vi "Import - Tx Packet.vi"(7 "Tx Packet":T1 {"Endianness" items=["big-endian"=0, "little-endian"=2]}, 8 "error in (no error)":errorcluster, 11 "Device Item Ref in":T6 format="%.0x") -> (0 "error out":errorcluster)   [LabVIEW 2016, in "UDP-Custom-Device System Explorer.lvlib"]
uses:
  UDP-Custom-Device System Explorer.lvlib
  <vilib>/NI Veristand/Custom Device API/Custom Device Item Ref.ctl
  Types/XML - New/ImpExp - Tx Packet Data.ctl
  <vilib>/NI Veristand/Custom Device API/Custom Device Item Info.ctl
  Shared/Types/Shared - Channel Data Type.ctl
  Shared/Types/Shared - Buffered.PacketInfo.ctl
  Shared/Types/Shared - Pointer Encoding.ctl
  Property Accessors/Shared Packet Accessors.lvlib
  Property Accessors/Tx Packet Accessors.lvlib
  <vilib>/NI VeriStand/Custom Device API/Custom Device API.lvlib
  <vilib>/NI VeriStand/Custom Device Tools/Custom Device Utility Library/Custom Device Utility Library.lvlib
  Shared/UDP-Custom-Device Shared.lvlib
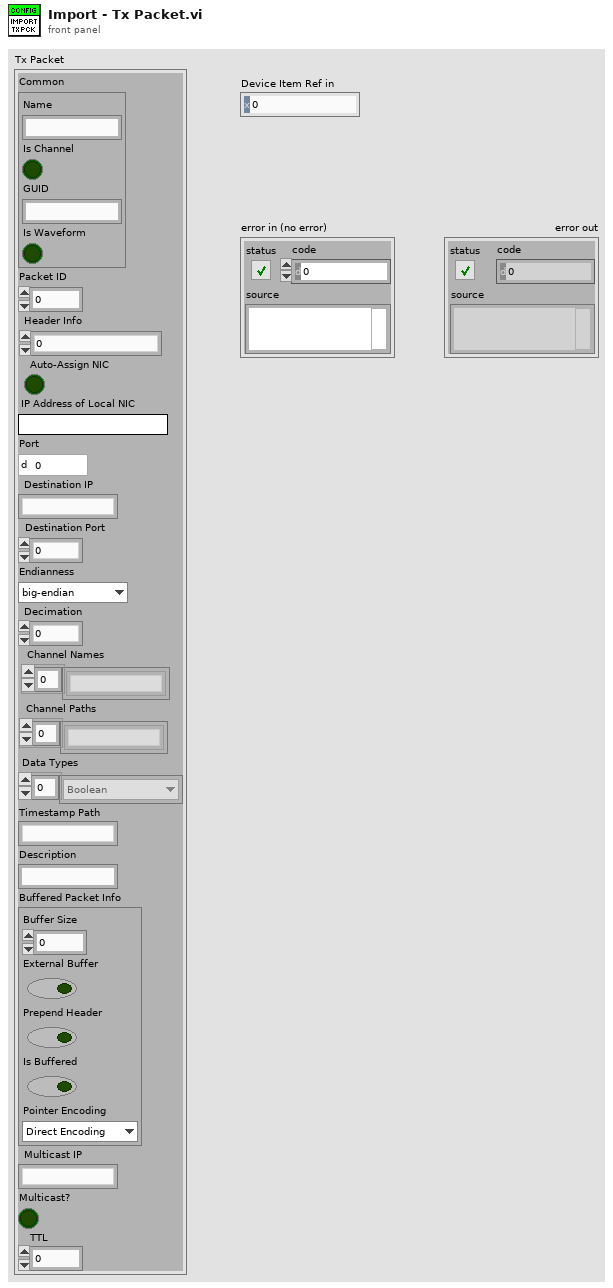
[diagram p1: front panel]
types:
  T1 = typedef "UDP-Custom-Device System Explorer.lvlib/ImpExp - Tx Packet Data.ctl" = cluster{"Common":T2, "Packet ID":i32, "Header Info":u32, "Auto-Assign NIC":bool, "IP Address of Local NIC":string, "Port":u16, "Destination IP":string, "Destination Port":u16, "Endianness":u16, "Decimation":u16, "Channel Names":string[], "Channel Paths":string[], "Data Types":T3[], "Timestamp Path":string, "Description":string, "Buffered Packet Info":T4, "Multicast IP":string, "Multicast?":bool, "TTL":u16}
  T2 = typedef "Custom Device API.lvlib/Custom Device Item Info.ctl" = cluster{"Name":string, "Is Channel":bool, "GUID":string, "Is Waveform":bool}
  T3 = typedef "UDP-Custom-Device Shared.lvlib/Shared - Channel Data Type.ctl" = enum16{"Boolean", "Single", "Double", "I8", "I16", "I32", "I64", "U8", "U16", "U32", "U64"}
  T4 = typedef "UDP-Custom-Device Shared.lvlib/Shared - Buffered.PacketInfo.ctl" = cluster{"Buffer Size":i32, "External Buffer":bool, "Prepend Header":bool, "Is Buffered":bool, "Pointer Encoding":T5}
  T5 = typedef "UDP-Custom-Device Shared.lvlib/Shared - Pointer Encoding.ctl" = enum16{"Direct Encoding", "Conversion Encoding"}
  T6 = typedef "Custom Device API.lvlib/Custom Device Item Ref.ctl" = u64
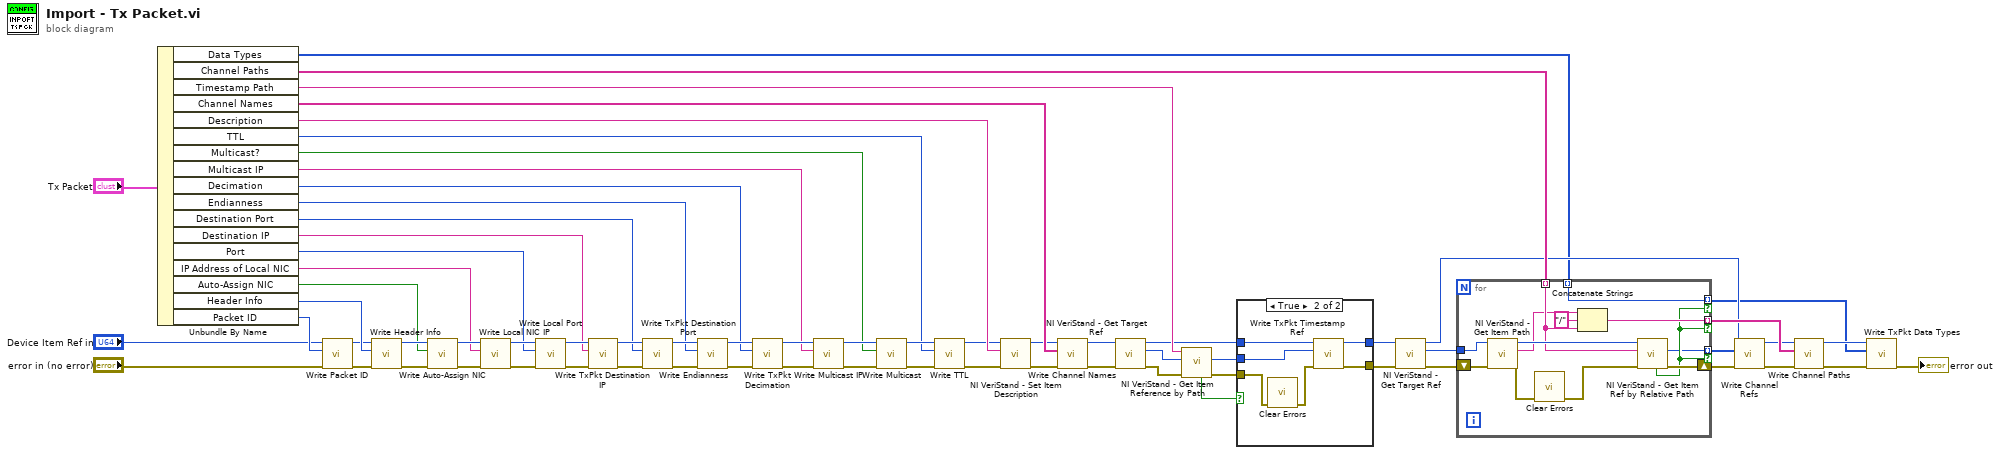
[diagram p0: block diagram]
diagram:
  n1 = Unbundle By Name("Tx Packet") -> ("Data Types"=w16:T3[], "Channel Paths"=w24:string[], "Timestamp Path"=w31:string, "Channel Names"=w39:string[], "Description"=w42:string, "TTL"=w1:u16, "Multicast?"=w2:bool, "Multicast IP"=w3:string, "Decimation"=w43:u16, "Endianness"=w44:u16, "Destination Port"=w49:u16, "Destination IP"=w50:string, "Port"=w51:u16, "IP Address of Local NIC"=w52:string, "Auto-Assign NIC"=w61:bool, "Header Info"=w66:u32, "Packet ID"=w67:i32)
  n2 = call "Write Packet ID.vi"("error in (no error)"="error in (no error)", "Packet ID"=w67, "Node Ptr"="Device Item Ref in") -> ("error out"=w64:errorcluster, "Node Ptr out"=w65:T6)  [unwired: 7 in]
  n3 = call "Write Header Info.vi"("error in (no error)"=w64, "Header Info"=w66, "Node Ptr"=w65) -> ("error out"=w62:errorcluster, "Node Ptr out"=w63:T6)  [unwired: 7 in]
  n4 = call "Write Auto-Assign NIC.vi"("error in (no error)"=w62, "Auto-Assign NIC"=w61, "Node Ptr"=w63) -> ("error out"=w56:errorcluster, "Node Ptr out"=w60:T6)  [unwired: 7 in]
  n5 = call "Write Local NIC IP.vi"("error in (no error)"=w56, "IP Address of Local NIC"=w52, "Node Ptr"=w60) -> ("error out"=w55:errorcluster, "Node Ptr out"=w59:T6)  [unwired: 7 in]
  n6 = call "Write Local Port.vi"("error in (no error)"=w55, "Port"=w51, "Node Ptr"=w59) -> ("error out"=w54:errorcluster, "Node Ptr out"=w58:T6)  [unwired: 7 in]
  n7 = call "Write TxPkt Destination IP.vi"("error in (no error)"=w54, "Destination IP"=w50, "Node Ptr"=w58) -> ("error out"=w53:errorcluster, "Node Ptr out"=w57:T6)  [unwired: 7 in]
  n8 = call "Write TxPkt Destination Port.vi"("error in (no error)"=w53, "Destination Port"=w49, "Node Ptr"=w57) -> ("error out"=w47:errorcluster, "Node Ptr out"=w48:T6)  [unwired: 7 in]
  n9 = call "Write Endianness.vi"("error in (no error)"=w47, "Endianness"=w44, "Node Ptr"=w48) -> ("error out"=w45:errorcluster, "Node Ptr out"=w46:T6)  [unwired: 7 in]
  n10 = call "Write TxPkt Decimation.vi"("error in (no error)"=w45, "Decimation"=w43, "Node Ptr"=w46) -> ("error out"=w11:errorcluster, "Node Ptr out"=w5:T6)  [unwired: 7 in]
  n11 = call "Write Multicast IP.vi"("error in (no error)"=w11, "Multicast IP Address"=w3, "Node Ptr"=w5) -> ("error out"=w10:errorcluster, "Node Ptr out"=w7:T6)  [unwired: 7 in]
  n12 = call "Write Multicast.vi"("error in (no error)"=w10, "Multicast"=w2, "Node Ptr"=w7) -> ("error out"=w9:errorcluster, "Node Ptr out"=w6:T6)  [unwired: 7 in]
  n13 = call "Write TTL.vi"("error in (no error)"=w9, "TTL"=w1, "Node Ptr"=w6) -> ("error out"=w8:errorcluster, "Node Ptr out"=w4:T6)  [unwired: 7 in]
  n14 = call <vilib>:"NI VeriStand - Set Item Description.vi"("error in (no error)"=w8, "Description"=w42, "Item Ref in"=w4) -> ("error out"=w37:errorcluster, "Item Ref out"=w38:T6)  [unwired: 6 in, 1 out]
  n15 = call "Write Channel Names.vi"("error in (no error)"=w37, "Channel Names"=w39, "Node Ptr"=w38) -> ("error out"=w32:errorcluster, "Node Ptr out"=w33:T6)  [unwired: 7 in]
  n16 = call <vilib>:"NI VeriStand - Get Target Ref.vi"("error in"=w32, "Item Ref in"=w33) -> ("error out"=w35:errorcluster, "Target Ref"=w36:T6, "Item Ref out"=w30:T6)  [unwired: 6 in, 1 out]
  n17 = call <vilib>:"NI VeriStand - Get Item Reference by Path.vi"("error in (no error)"=w35, "Root Ref"=w36, "Item Path in"=w31) -> ("error out"=w34:errorcluster, "Item Ref"=w29:T6, "Found"=w22:bool)  [unwired: 5 in, 1 out]
  n18 = case shown="True" w22 {
    tunnel: w34 -> [w69 w76]
    tunnel: w30 -> [w70 w75]
    tunnel: w29 -> [_ w74]
    tunnel: [w70 w72] -> w28
    tunnel: [w69 w71] -> w27
    frame False {
    }
    frame True {
      n19 = call <vilib>:"Clear Errors.vi"("error in (no error)"=w76) -> ("error out"=w73:errorcluster)  [unwired: 5 in, 1 out]
      n20 = call "Write TxPkt Timestamp Ref.vi"("error in (no error)"=w73, "Dependent Node Ref"=w74, "Node Ptr"=w75) -> ("error out"=w71:errorcluster, "Node Ptr out"=w72:T6)  [unwired: 7 in]
    }
  }
  n21 = call <vilib>:"NI VeriStand - Get Target Ref.vi"("error in"=w27, "Item Ref in"=w28) -> ("error out"=w25:errorcluster, "Target Ref"=w26:T6, "Item Ref out"=w20:T6)  [unwired: 6 in, 1 out]
  n22 = for {
    tunnel: w26 -> [w89]
    tunnel: w24 -> [w79] mode=indexing
    tunnel: [w85] -> w23 mode=indexing if=w81
    tunnel: [w80] -> w21 mode=indexing if=w81
    shift-right: [w82] -> w17
    shift-left: w25 -> [w88]
    tunnel: w16 -> [w86] mode=indexing
    tunnel: [w86] -> w12 mode=indexing if=w81
    n23 = call <vilib>:"NI VeriStand - Get Item Path.vi"("error in (no error)"=w88, "Item Ref in"=w89) -> ("error out"=w87:errorcluster, "Path"=w78:string, "Item Ref out"=w84:T6)  [unwired: 6 in, 1 out]
    n24 = call <vilib>:"Clear Errors.vi"("error in (no error)"=w87) -> ("error out"=w83:errorcluster)  [unwired: 5 in, 1 out]
    n25 = Concatenate Strings(w78, "/" ("string"), w79) -> (w85:string)
    n26 = call <vilib>:"NI VeriStand - Get Item Ref by Relative Path.vi"("error in"=w83, "Relative Item Path"=w79, "Section Ref in"=w84) -> ("error out"=w82:errorcluster, "Item Ref"=w80:T6, "Found"=w81:bool)  [unwired: 5 in, 1 out]
  }
  n27 = call "Write Channel Refs.vi"("error in (no error)"=w17, "Dependent Node Refs"=w21, "Node Ptr"=w20) -> ("error out"=w18:errorcluster, "Node Ptr out"=w19:T6)  [unwired: 7 in]
  n28 = call "Write Channel Paths.vi"("error in (no error)"=w18, "Channel Paths"=w23, "Node Ptr"=w19) -> ("error out"=w15:errorcluster, "Node Ptr out"=w13:T6)  [unwired: 7 in]
  n29 = call "Write TxPkt Data Types.vi"("error in (no error)"=w15, "Data Types"=w12, "Node Ptr"=w13) -> ("error out"=→"error out":errorcluster)  [unwired: 7 in, 1 out]
